vi "Test My Singleton Module API.vi"() -> ()   [LabVIEW 2019]
doc: "My Singleton Module API Tester.\n_____\nBased on Delacor QMH Project Template 4.2.1.64."
uses:
  My Singleton Module.lvlib
panel:
  in  "wait for reply":bool=TRUE
  in  "Show Block Diagram":bool
  in  "X":dbl=1.0
  out "Reply Payload":dbl
  in  "Stop Module":bool
  in  "Start Module":bool
  out "Do Something Count":i32
  in  "Test Do Something Else and Wait for Reply":bool
  in  "Hide Module Panel":bool
  in  "Show Module Panel":bool
  in  "Test Do Something Else":bool
  in  "Test Do Something":bool
  out "Status":string
  out "Module Running?":bool
  # "This VI tests the API for the Module."
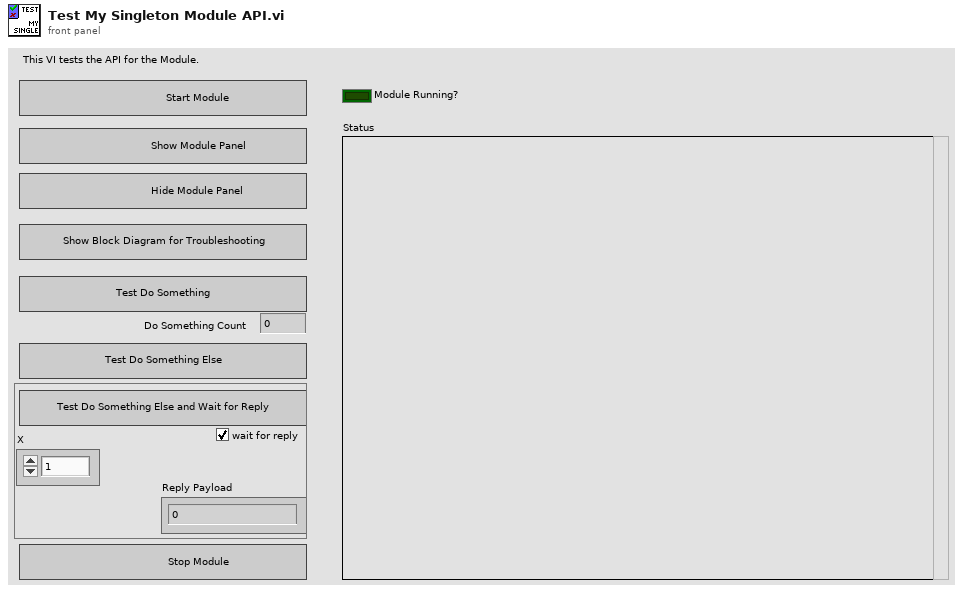
[diagram p1: front panel]
types:
  T1 = typedef "My Singleton Module.lvlib/Broadcast Events--cluster.ctl" = cluster{"Module Did Init":refnum<user-event>, "Status Updated":refnum<user-event>, "Error Reported":refnum<user-event>, "Did Something":refnum<user-event>, "Module Did Stop":refnum<user-event>, "Update Module Execution Status":refnum<user-event>}
  T2 = typedef "My Singleton Module.lvlib/Do Something Else and Wait (Reply Payload)--cluster.ctl" = cluster{"Value":dbl, "error":errorcluster}
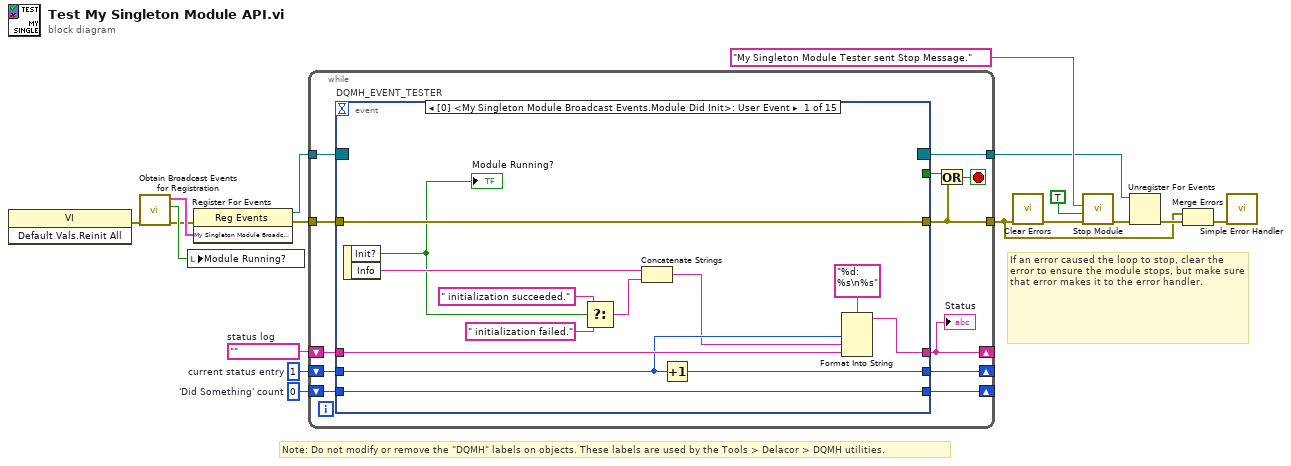
[diagram p0: block diagram]
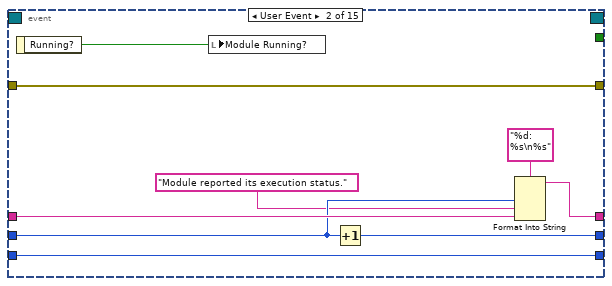
[diagram p2: hidden frame]
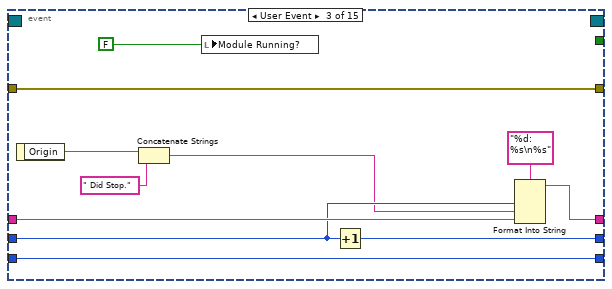
[diagram p3: hidden frame]
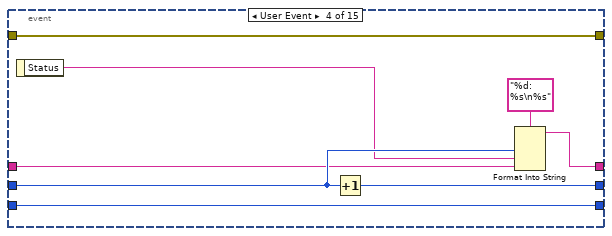
[diagram p4: hidden frame]
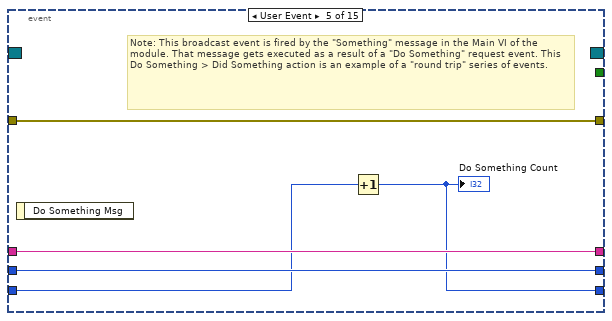
[diagram p5: hidden frame]
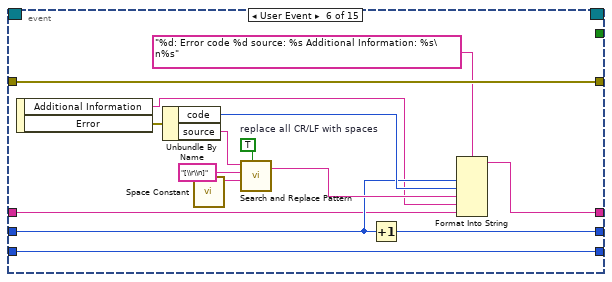
[diagram p6: hidden frame]
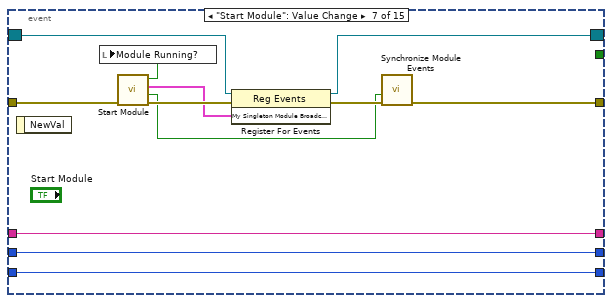
[diagram p7: hidden frame]
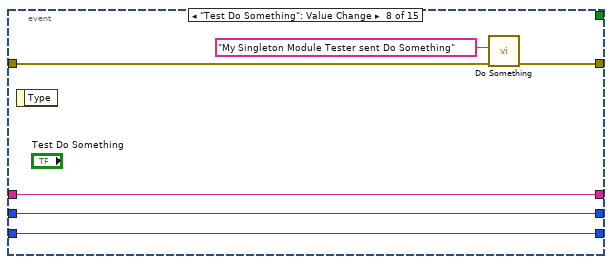
[diagram p8: hidden frame]
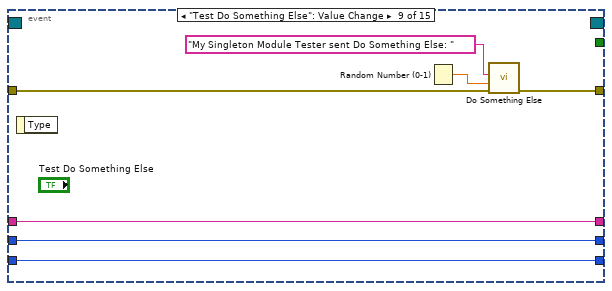
[diagram p9: hidden frame]
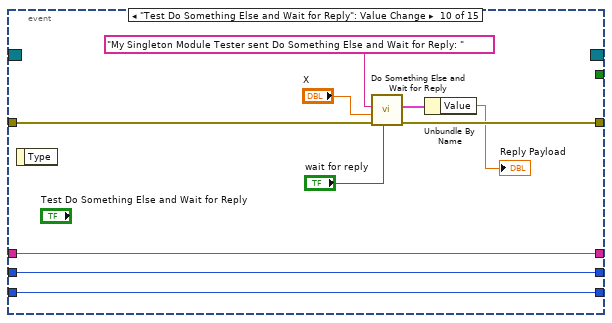
[diagram p10: hidden frame]
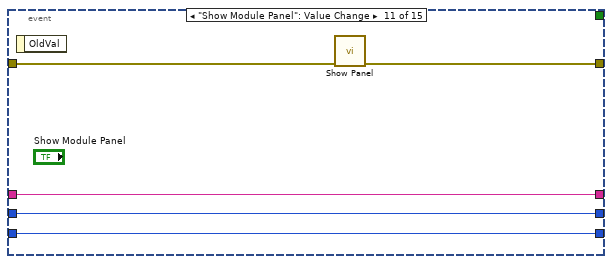
[diagram p11: hidden frame]
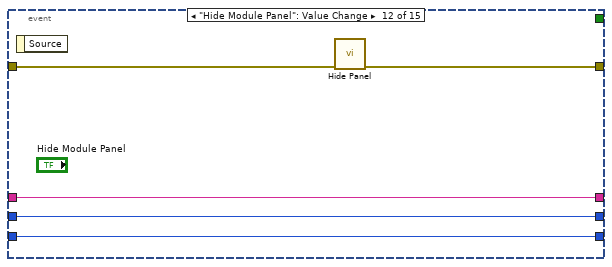
[diagram p12: hidden frame]
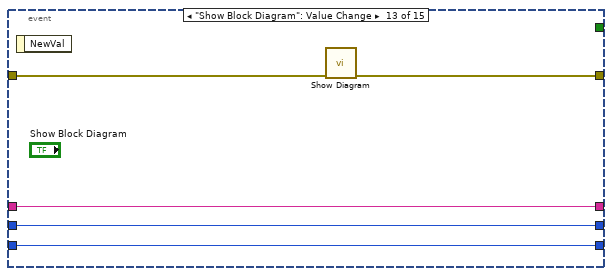
[diagram p13: hidden frame]
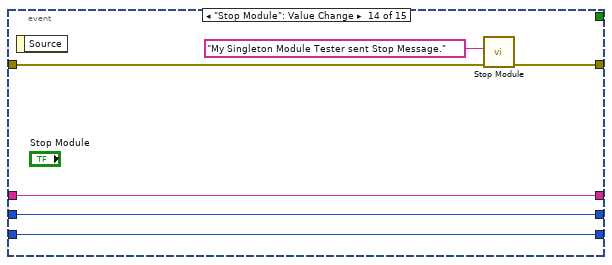
[diagram p14: hidden frame]
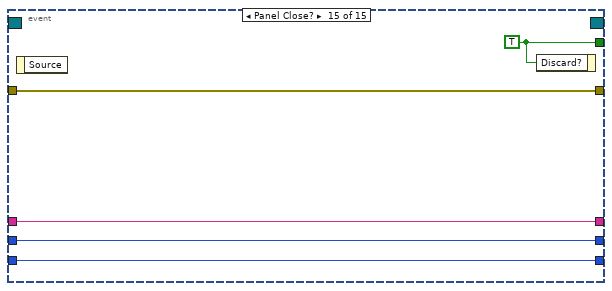
[diagram p15: hidden frame]
diagram:
  w12 = 0  # 'Did Something' count
  w13 = 1  # current status entry
  w14 = ""  # status log
  # "If an error caused the loop to stop, clear the error to ensure the module stops, but make sure that error makes it to the error handler."
  # "Note: Do not modify or remove the \"DQMH\" labels on objects. These labels are used by the Tools > Delacor > DQMH utilities."
  n1 = invoke class="VI" method="Default Vals.Reinit All"() -> (error out=w2:errorcluster)  [unwired: 3 in, 2 out]
  n2 = call "Obtain Broadcast Events for Registration.vi"("error in (no error)"=w2) -> ("error out"=w1:errorcluster, "Already running?"=w3:bool, "My Singleton Module Broadcast Events"=w10:T1)  [unwired: 8 in]
  n3 = local write "Module Running?"(w3) -> ()
  n4 = register-events(error in=w1, w10) -> (reference out=w9:refnum<event-registration>, error out=w11:errorcluster)  [unwired: 1 in]
  n5 = while {
    tunnel: w9 -> [w29]
    tunnel: [w18] -> w4
    shift-right: [w24] -> _
    shift-left: w14 -> [w26]
    shift-right: [w25] -> _
    shift-left: w13 -> [w27]
    shift-right: [w22] -> _
    shift-left: w12 -> [w23]
    tunnel: w11 -> [w20]
    tunnel: [w19] -> w8
    stop <- w21 stop-if-true
    n6 = event "DQMH_EVENT_TESTER" shown="[0] <My Singleton Module Broadcast Events.Module Did Init>: User Event" {
      selector: w29 -> [_ _ _ _ _ _ w95 _ _ _ _ _ _ _ _]
      dyn-events: [_ _ _ _ _ _ w94 _ _ _ _ _ _ _ _] -> w19
      timeout: _ -> [_ _ _ _ _ _ _ _ _ _ _ _ _ _ _]
      tunnel: [_ _ _ _ _ _ _ _ _ _ _ _ _ _ w151] -> w28
      tunnel: [w42 w44 w52 w63 w71 w89 w93 w108 w115 w125 w130 w135 w136 w143 w147] -> w18
      tunnel: w27 -> [w39 w49 w60 w67 w74 w79 w99 w105 w111 w122 w128 w133 w138 w145 w149]
      tunnel: w26 -> [w40 w50 w61 w66 w75 w77 w100 w106 w112 w123 w129 w134 w139 w146 w150]
      tunnel: [w37 w47 w58 w68 w75 w80 w100 w106 w112 w123 w129 w134 w139 w146 w150] -> w24
      tunnel: [w38 w48 w59 w70 w74 w78 w99 w105 w111 w122 w128 w133 w138 w145 w149] -> w25
      tunnel: w23 -> [w34 w45 w54 w64 w73 w90 w98 w104 w110 w121 w127 w132 w137 w144 w148]
      tunnel: [w34 w45 w54 w64 w72 w90 w98 w104 w110 w121 w127 w132 w137 w144 w148] -> w22
      tunnel: w20 -> [w42 w44 w52 w63 w71 w89 w92 w103 w109 w118 w126 w131 w140 w141 w147]
      event User Event {
        n7 = event-data() -> ("Init?"=w33:bool, "Info"=w36:string)  [unwired: 1 in]
        "Module Running?" <- w33
        n8 = Select(t=" initialization succeeded.", s=w33, f=" initialization failed.") -> (s? t:f=w30:string)
        n9 = Concatenate Strings(w36, w30) -> (w35:string)
        n10 = Increment(x=w39) -> (x+1=w38:i32)
        n11 = Format Into String(format string="%d: %s\n%s", w39, w35, w40) -> (resulting string=w37:string)  [unwired: 2 in, 1 out]
      }
      event User Event {
        n12 = event-data() -> ("Running?"=w43:bool)  [unwired: 1 in]
        n13 = local write "Module Running?"(w43) -> ()
        n14 = Increment(x=w49) -> (x+1=w48:i32)
        n15 = Format Into String(format string="%d: %s\n%s", w49, "Module reported its execution status.", w50) -> (resulting string=w47:string)  [unwired: 2 in, 1 out]
      }
      event User Event {
        n16 = event-data() -> ("Origin"=w57:string)  [unwired: 1 in]
        n17 = Concatenate Strings(w57, " Did Stop.") -> (w56:string)
        n18 = local write "Module Running?"(FALSE ("Module Did Init?")) -> ()
        n19 = Increment(x=w60) -> (x+1=w59:i32)
        n20 = Format Into String(format string="%d: %s\n%s", w60, w56, w61) -> (resulting string=w58:string)  [unwired: 2 in, 1 out]
      }
      event User Event {
        n21 = event-data() -> ("Status"=w65:string)  [unwired: 1 in]
        n22 = Increment(x=w67) -> (x+1=w70:i32)
        n23 = Format Into String(format string="%d: %s\n%s", w67, w65, w66) -> (resulting string=w68:string)  [unwired: 2 in, 1 out]
      }
      event User Event {
        # "Note: This broadcast event is fired by the \"Something\" message in the Main VI of the module. That message gets executed as a result of a \"Do Something\" request event. This Do Something > Did Something action is an example of a \"round trip\" series of events."
        n24 = event-data() -> ()  [unwired: 1 in, 1 out]
        n25 = Increment(x=w73) -> (x+1=w72:i32)
        "Do Something Count" <- w72
      }
      event User Event {
        w85 = TRUE  # replace all CR/LF with spaces
        n26 = event-data() -> ("Additional Information"=w76:string, "Error"=w81:errorcluster)  [unwired: 1 in]
        n27 = Unbundle By Name(w81) -> ("code"=w82:i32, "source"=w83:string)
        n28 = call <vilib>:"Space Constant.vi"() -> ("String"=w86:string)
        n29 = call <vilib>:"Search and Replace Pattern.vi"("string"=w83, "regular expression (\"\")"="[\\r\\n]" ("regular expression (\"\")"), "replace string (\"\")"=w86, "replace all? (F)"=w85) -> ("result string"=w84:string)  [unwired: 1 in, 1 out]
        n30 = Increment(x=w79) -> (x+1=w78:i32)
        n31 = Format Into String(format string="%d: Error code %d source: %s Additional Information: %s\n%s", w79, w82, w84, w76, w77) -> (resulting string=w80:string)  [unwired: 2 in, 1 out]
      }
      event "Start Module": Value Change {
        n32 = event-data() -> ()  [unwired: 1 in, 1 out]
        n33 = call "Start Module.vi"("error in (no error)"=w92) -> ("error out"=w101:errorcluster, "Wait for Event Sync?"=w97:bool, "My Singleton Module Broadcast Events"=w96:T1, "Module Was Already Running?"=w91:bool)  [unwired: 7 in]
        n34 = local write "Module Running?"(w91) -> ()
        n35 = register-events(reference=w95, error in=w101, w96) -> (reference out=w94:refnum<event-registration>, error out=w102:errorcluster)
        n36 = call "Synchronize Module Events.vi"("error in (no error)"=w102, "Wait for Event Sync?"=w97) -> ("error out"=w93:errorcluster)  [unwired: 9 in]
      }
      event "Test Do Something": Value Change {
        n37 = event-data() -> ()  [unwired: 1 in, 1 out]
        n38 = call "Do Something.vi"("error in (no error)"=w103, "Do Something Message"="My Singleton Module Tester sent Do Something") -> ("error out"=w108:errorcluster)  [unwired: 9 in]
      }
      event "Test Do Something Else": Value Change {
        n39 = event-data() -> ()  [unwired: 1 in, 1 out]
        n40 = Random Number (0-1)() -> (number: 0 to 1=w113:dbl)
        n41 = call "Do Something Else.vi"("error in (no error)"=w109, "X"=w113, "Do Something Else Message"="My Singleton Module Tester sent Do Something Else: " ("Do Something Message")) -> ("error out"=w115:errorcluster)  [unwired: 8 in]
      }
      event "Test Do Something Else and Wait for Reply": Value Change {
        n42 = event-data() -> ()  [unwired: 1 in, 1 out]
        n43 = call "Do Something Else and Wait for Reply.vi"("wait for reply (T)"="wait for reply", "error in (no error)"=w118, "X"="X", "Do Something Else Message"="My Singleton Module Tester sent Do Something Else and Wait for Reply: " ("Do Something Message")) -> ("error out"=w125:errorcluster, "Reply Payload"=w120:T2)  [unwired: 5 in, 1 out]
        n44 = Unbundle By Name(w120) -> ("Value"=→"Reply Payload":dbl)
      }
      event "Show Module Panel": Value Change {
        n45 = event-data() -> ()  [unwired: 1 in, 1 out]
        n46 = call "Show Panel.vi"("error in (no error)"=w126) -> ("error out"=w130:errorcluster)  [unwired: 10 in]
      }
      event "Hide Module Panel": Value Change {
        n47 = event-data() -> ()  [unwired: 1 in, 1 out]
        n48 = call "Hide Panel.vi"("error in (no error)"=w131) -> ("error out"=w135:errorcluster)  [unwired: 10 in]
      }
      event "Show Block Diagram": Value Change {
        n49 = event-data() -> ()  [unwired: 1 in, 1 out]
        n50 = call "Show Diagram.vi"("error in (no error)"=w140) -> ("error out"=w136:errorcluster)  [unwired: 10 in]
      }
      event "Stop Module": Value Change {
        n51 = event-data() -> ()  [unwired: 1 in, 1 out]
        n52 = call "Stop Module.vi"("error in (no error)"=w141, "Origin"="My Singleton Module Tester sent Stop Message.") -> ("error out"=w143:errorcluster)  [unwired: 9 in]
      }
      event Panel Close? {
        w151 = TRUE ("Discard?")
        n53 = event-data() -> ()  [unwired: 1 in, 1 out]
        n54 = event-data("Discard?"=w151) -> ()  [unwired: 1 in, 1 out]
      }
    }
    "Status" <- w24
    n55 = Or(x=w28, y=w18) -> (x .or. y?=w21:bool)
  }
  n56 = call <vilib>:"Clear Errors.vi"("error in (no error)"=w4) -> ("error out"=w6:errorcluster)  [unwired: 5 in, 1 out]
  n57 = call "Stop Module.vi"("error in (no error)"=w6, "Wait for Module to Stop? (F)"=TRUE ("Wait for Module to stop?"), "Origin"="My Singleton Module Tester sent Stop Message.") -> ("error out"=w16:errorcluster)  [unwired: 8 in]
  n58 = Unregister For Events(event registration refnum=w8, error in=w16) -> (error out=w17:errorcluster)
  n59 = Merge Errors(w4, w17) -> (w5:errorcluster)
  n60 = call <vilib>:"Simple Error Handler.vi"("error in (no error)"=w5) -> ()  [unwired: 4 in, 5 out]
